vi "find devices.vi"() -> ()   [LabVIEW 2013, in "libusvlv.lvlib"]
uses:
  libusvlv.lvlib
  UsbCom.dll
panel:
  out "pid":i32 format="%x"
  out "vid":i32 format="%x"
  out "devices":i32
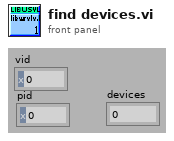
[diagram p1: front panel]
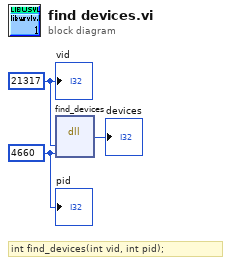
[diagram p0: block diagram]
diagram:
  w2 = 4660
  w3 = 21317
  # "int find_devices(int vid, int pid);"
  n1 = dll-call lib="E:/libusvlv/UsbCom.dll" fn="find_devices"("vid"=w3, "pid"=w2) -> ("num"=→"devices":i32)  [unwired: 5 in, 2 out]
  "vid" <- w3
  "pid" <- w2
